vi "Compute_Fit.vi"(4 "timeout":i32=30000, 5 "clip":dbl, 6 "binsize":i32, 7 "error in":errorcluster, 8 "fit_function":string="Gaussian", 9 "data":sgl[][](array[numeric]), 10 "context in":refnum<class "zmq_context.lvclass">) -> (0 "error out":errorcluster, 1 "Y_section":dbl[][](array[numeric]), 2 "X_section":dbl[][](array[numeric]), 3 "fit":variant)   [LabVIEW 2010]
uses:
  <vilib>/addons/zeromq/zmq_context.lvclass
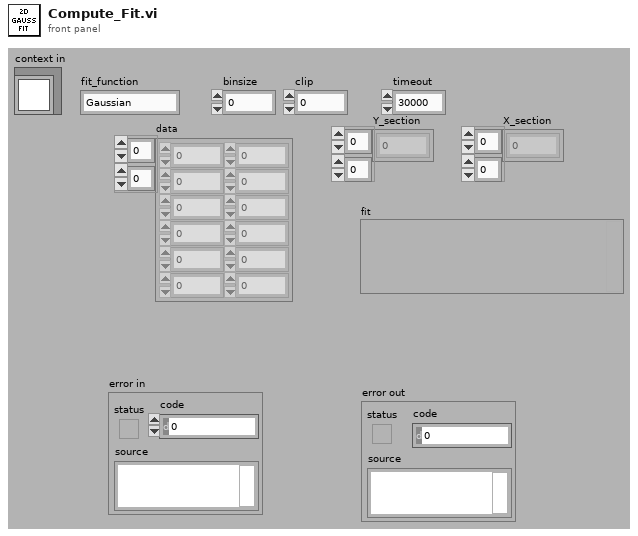
[diagram p1: front panel]
types:
  T1 = cluster{"fit_function":string, "binsize":i32, "clip":dbl}
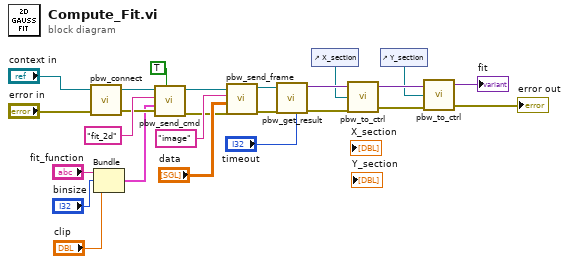
[diagram p0: block diagram]
diagram:
  n1 = call <vilib>:"pbw_connect.vi"("error in"="error in", "context in"="context in") -> ("error out"=w9:errorcluster, "socket out"=w22:refnum<class "zmq_socket.lvclass">)  [unwired: 2 in]
  n2 = Bundle("fit_function"="fit_function", "binsize"="binsize", "clip"="clip") -> (w8:T1)  [unwired: 1 in]
  n3 = call <vilib>:"pbw_send_cmd.vi"("more? (F)"=TRUE, "error in"=w9, "cluster"=w8, "command"="fit_2d" ("data"), "socket in"=w22) -> ("error out"=w6:errorcluster, "socket out"=w7:refnum<class "zmq_socket.lvclass">)  [unwired: 2 in]
  n4 = call <vilib>:"pbw_send_frame.vi"("error in"=w6, "data"="data", "name"="image", "socket in"=w7) -> ("error out"=w4:errorcluster, "socket out"=w5:refnum<class "zmq_socket.lvclass">)  [unwired: 3 in]
  n5 = call <vilib>:"pbw_get_result.vi"("error in"=w4, "socket in"=w5, "timeout"="timeout") -> ("error out"=w15:errorcluster, "return vals"=w17:variant)  [unwired: 4 in]
  n6 = control-ref of="X_section"() -> (w16:refnum<vi>)
  n7 = call <vilib>:"pbw_to_ctrl.vi"("error in"=w15, "control"=w16, "variant w attribs"=w17) -> ("error out"=w13:errorcluster, "duplicate variant"=w14:variant)  [unwired: 1 out]
  n8 = control-ref of="Y_section"() -> (w12:refnum<vi>)
  n9 = call <vilib>:"pbw_to_ctrl.vi"("error in"=w13, "control"=w12, "variant w attribs"=w14) -> ("error out"=→"error out":errorcluster, "duplicate variant"=→"fit":variant)  [unwired: 1 out]
